vi "setT7Inclinometer.vi"(10 "T7Inclinometer":refnum<class "T7Inclinometer.lvclass">, 11 "Model in":refnum<class "Model.lvclass">) -> (3 "Model out":refnum<class "Model.lvclass">)   [LabVIEW 2016, in "Model.lvclass"]
uses:
  Model.lvclass
  Common_RT_T7Inclinometer/T7Inclinometer/T7Inclinometer.lvclass
  Model.lvclass/Model.ctl
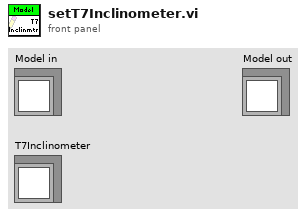
[diagram p1: front panel]
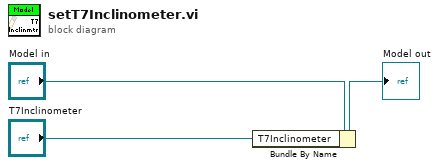
[diagram p0: block diagram]
diagram:
  n1 = Bundle By Name(cluster="Model in", "T7Inclinometer"="T7Inclinometer") -> (→"Model out":refnum<class "Model.lvclass">)
